vi "manual-induction-furnace-control-v5.vi"() -> ()   [LabVIEW 2019]
uses:
  <vilib>/DAQmx/read.llb/DAQmx Read (Analog 2D DBL NChan NSamp).vi
  <vilib>/Analysis/baseanly.llb/Mean (DBL).vi
  <vilib>/DAQmx/read.llb/DAQmx Read (Analog 1D DBL 1Chan NSamp).vi
  <vilib>/DAQmx/write.llb/DAQmx Write (Analog DBL 1Chan 1Samp).vi
  <vilib>/DAQmx/create/channels.llb/DAQmx Create Channel (AO-Current-Basic).vi
  <vilib>/DAQmx/create/channels.llb/DAQmx Create Channel (AI-Current-Basic).vi
  <vilib>/DAQmx/create/channels.llb/DAQmx Create Channel (AI-Voltage-Basic).vi
  <vilib>/DAQmx/miscellaneous.llb/DAQmx Fill In Error Info.vi
  <vilib>/Analysis/NI_AALBase.lvlib
panel:
  out "Error Detected":bool
  in  "Furnace Enable":bool
  in  "Furnace Stop":bool
  out "Valve Output":dbl format="%#_3g"
  in  "ESTOP":bool
  in  "Valve Open":bool
  in  "Purge Flow On":bool
  out "Pressure":dbl format="%#_3g"
  in  "Tab Control":enum32{"Start", "Test", "End"}(tab)
  in  "Start Test":bool
  out "Waveform Chart":dynamicdata(graph)
  out "Test Elapsed Time":string
  in  "Stop / Reset":bool=TRUE caption="Start"
  in  "Data Log?":bool caption="Enable"
  in  "Data Collection Rate (10 hz max)":dbl=1.0 caption="Time Target (s)"
  in  "Pressure Limit (vacuum)":dbl=770.0
  in  "Temp change limit (per 0.5 sec)":dbl=60.0
  in  "Max Temp Limit":dbl=2600.0
  in  "Error Notification Recipient emails":string[](array[string])
  in  "Furnace Power":dbl min=0.0 max=100.0 step=0.1 format="%#.1f"
  in  "Argon Out":dbl format="%#_4g"
  in  "Auto ramp to 10%":bool
  in  "Heat-up rate":enum16{"Low", "Medium", "High"}(ring)
  in  "Filename":path=path "test.lvm"
  out "End Result":string
  out "Temperature":dbl format="%#_5g"
  out "Power Out":dbl
  # "%"
  # "°C"
  # "Torr"
  # "Check all of your hardware and setup, install your sample, turn on purge gas and pump down to your desired vacuum.\n\nClick the \"Start Test\" button when you are ready to start heating."
  # "This is a manual control window. Use the Auto Ramp button to get you to ~10%, then slowly increment the power percentage from 10% to your desired power while monitoring the temperature. Between each time you increment the power, allow enough time for the item in the furnace to come to equilibrium before increasing the power more."
  # "Manual Controls"
  # "%"
  # "%"
  # "Safety Shutoff Limits"
  # "Torr"
  # "°C"
  # "°C"
  # "Your test has been stopped. Below you can see if the test finished successfully or if an error occurred."
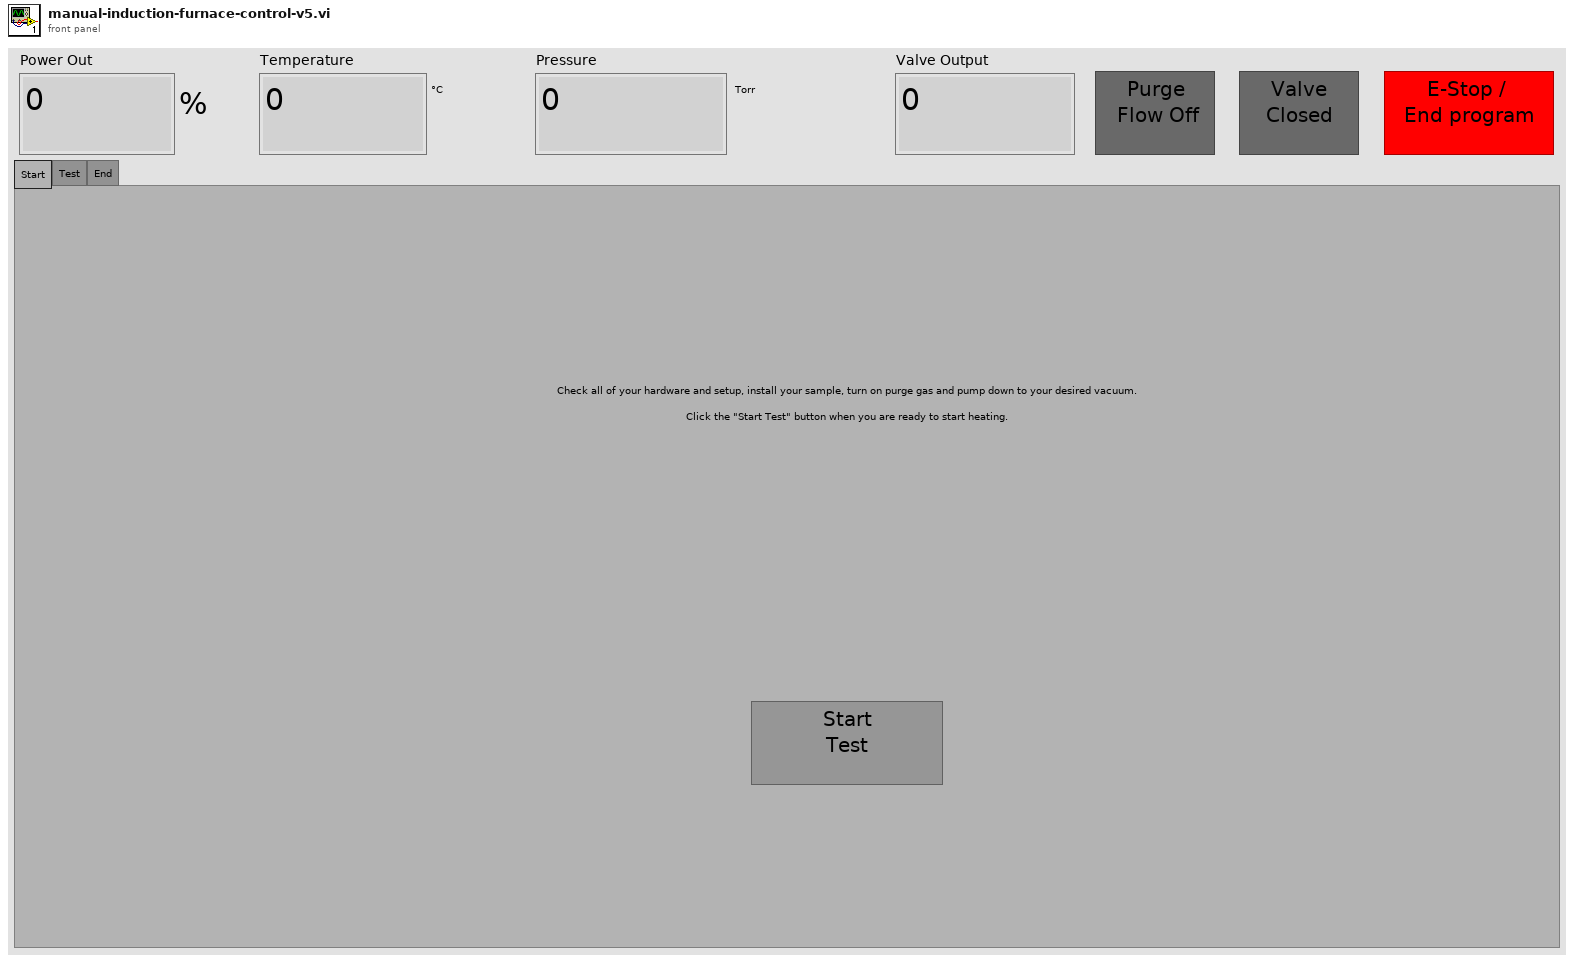
[diagram p1: front panel]
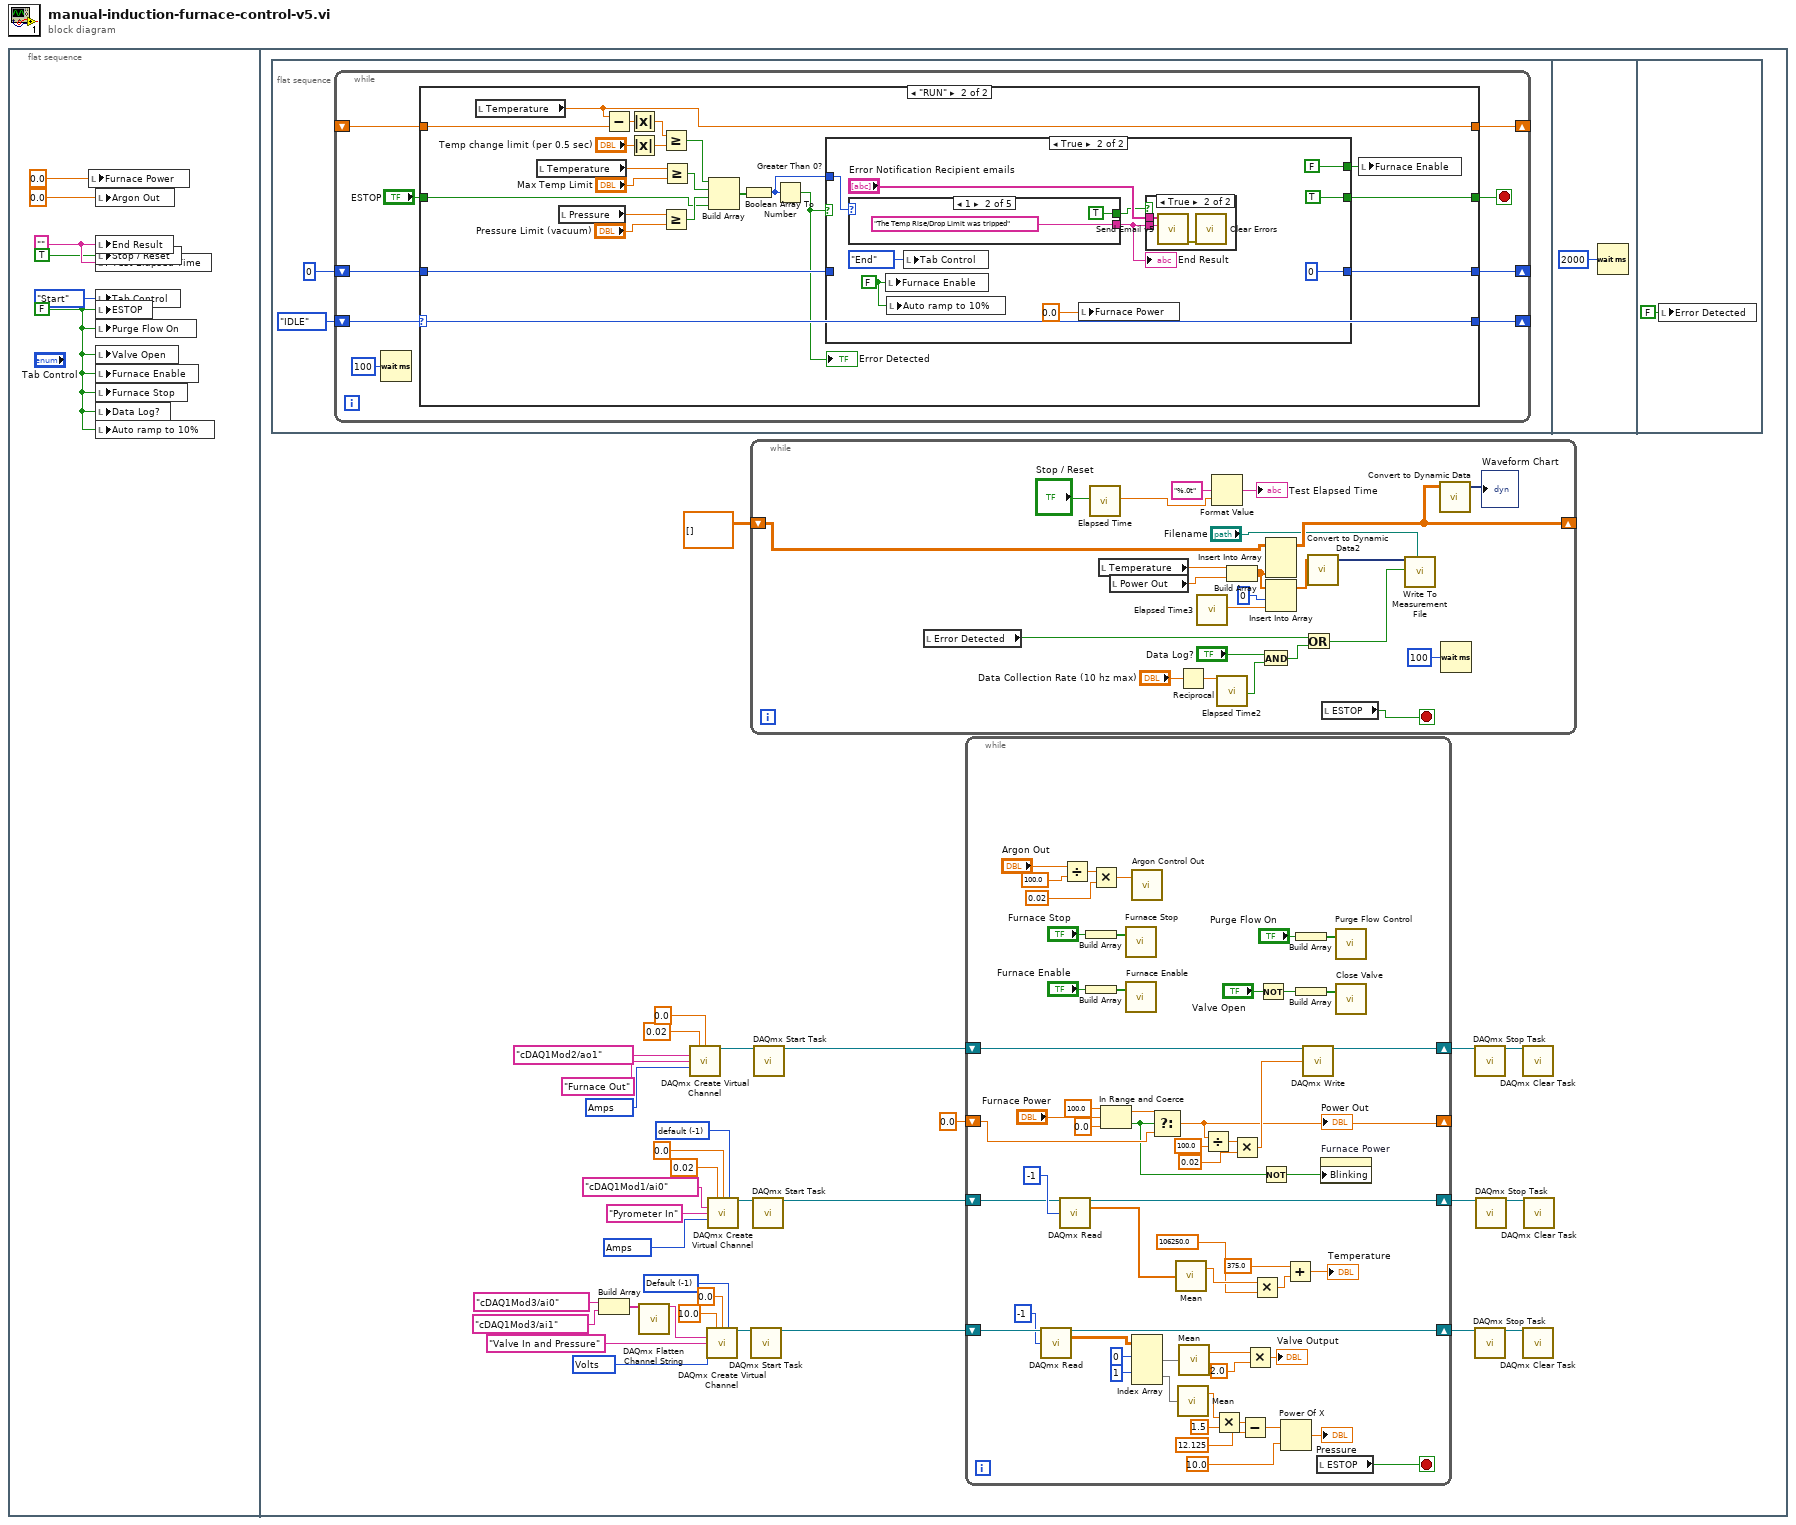
[diagram p0: block diagram]
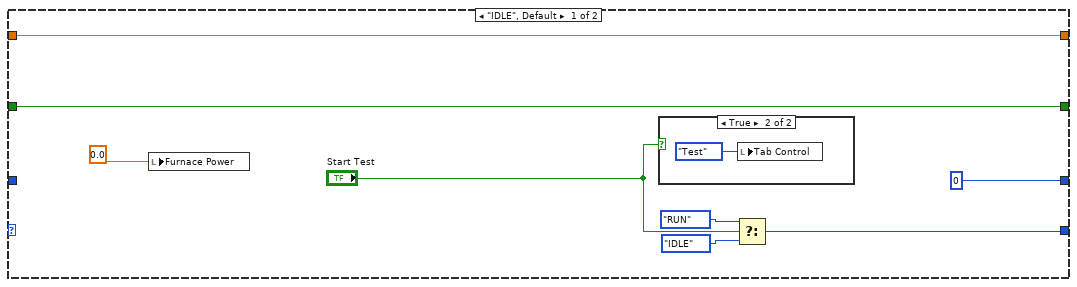
[diagram p2: hidden frame]
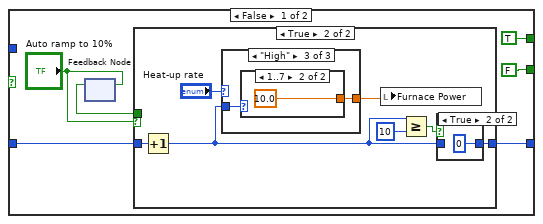
[diagram p4: hidden frame]
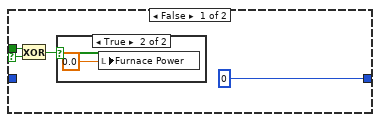
[diagram p5: hidden frame]
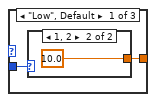
[diagram p7: hidden frame]
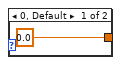
[diagram p8: hidden frame]
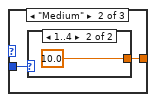
[diagram p9: hidden frame]
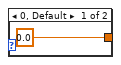
[diagram p10: hidden frame]
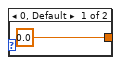
[diagram p11: hidden frame]
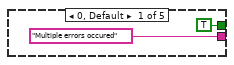
[diagram p14: hidden frame]
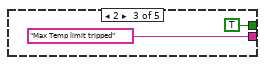
[diagram p15: hidden frame]
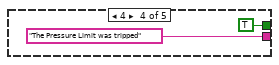
[diagram p16: hidden frame]
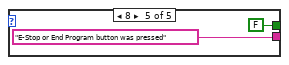
[diagram p17: hidden frame]
diagram:
  n1 = flat-sequence {
    frame #0 {
      w5 = "" ("End Result")
      w1 = FALSE
      n2 = local write "Furnace Power"(0.0 ("Power Input")) -> ()
      n3 = local write "Argon Out"(0.0 ("Pressure Limit")) -> ()
      n4 = local write "End Result"(w5) -> ()
      n5 = local write "Stop / Reset"(TRUE ("Stop / Reset")) -> ()
      n6 = local write "Test Elapsed Time"(w5) -> ()
      n7 = local write "Tab Control"(enum32{"Start", "Test", "End"}."Start" ("Tab Control")) -> ()
      n8 = local write "ESTOP"(w1) -> ()
      n9 = local write "Purge Flow On"(w1) -> ()
      n10 = local write "Valve Open"(w1) -> ()
      n11 = local write "Furnace Enable"(w1) -> ()
      n12 = local write "Furnace Stop"(w1) -> ()
      n13 = local write "Data Log?"(w1) -> ()
      n14 = local write "Auto ramp to 10%"(w1) -> ()
    }
    frame #1 {
      w20 = 10348 items=["Volts"=10348, "From Custom Scale"=10065] ("units")
      w22 = -1 items=["Default"=-1, "RSE"=10083, "NRSE"=10078, "Differential"=10106, "Pseudodifferential"=12529] ("input terminal configuration")
      w27 = -1 items=["default"=-1, "RSE"=10083, "NRSE"=10078, "Differential"=10106, "Pseudodifferential"=12529] ("input terminal configuration")
      w19 = 10342 items=["Amps"=10342, "From Custom Scale"=10065] ("units")
      w32 = 10342 items=["Amps"=10342, "From Custom Scale"=10065] ("units")
      n15 = flat-sequence {
        frame #0 {
          n16 = while {
            shift-right: [w47] -> _
            shift-left: enum16{"IDLE", "RUN"}."IDLE" -> [w49]
            shift-right: [w51] -> _
            shift-left: _ -> [w50]
            shift-right: [w45] -> _
            shift-left: 0 -> [w46]
            stop <- w43 stop-if-true
            n17 = Wait (ms)(milliseconds to wait=u32 100) -> ()  [unwired: 1 out]
            n18 = case shown="\"RUN\"" w49 {
              selector: w49 -> [_ w65]
              tunnel: [w59 w80] -> w51
              tunnel: w50 -> [w59 w79]
              tunnel: [w58 w66] -> w43
              tunnel: "ESTOP" -> [w58 w67]
              tunnel: [w55 w65] -> w47
              tunnel: w46 -> [_ w63]
              tunnel: [0 w62] -> w45
              frame "IDLE", Default {
                n19 = local write "Furnace Power"(0.0 ("Power Input")) -> ()
                n20 = case shown="True" "Start Test" {
                  frame False {
                  }
                  frame True {
                    n21 = local write "Tab Control"(enum32{"Start", "Test", "End"}."Test" ("Tab Control")) -> ()
                  }
                }
                n22 = Select(t=enum16{"IDLE", "RUN"}."RUN", s="Start Test", f=enum16{"IDLE", "RUN"}."IDLE") -> (s? t:f=w55:enum16{"IDLE", "RUN"})
              }
              frame "RUN" {
                n23 = local read "Temperature"() -> (w80:dbl)
                n24 = local read "Temperature"() -> (w74:dbl)
                n25 = local read "Pressure"() -> (w82:dbl)
                n26 = Subtract(x=w80, y=w79) -> (x-y=w76:dbl)
                n27 = Absolute Value(x=w76) -> (abs(x)=w75:dbl)
                n28 = Absolute Value(x="Temp change limit (per 0.5 sec)") -> (abs(x)=w77:dbl)
                n29 = Greater Or Equal?(x=w75, y=w77) -> (x >= y?=w72:bool)
                n30 = Greater Or Equal?(x=w82, y="Pressure Limit (vacuum)") -> (x >= y?=w70:bool)
                n31 = Greater Or Equal?(x=w74, y="Max Temp Limit") -> (x >= y?=w71:bool)
                n32 = Build Array(w72, w71, w70, w67) -> (w69:bool[])
                n33 = Boolean Array To Number(Boolean array=w69) -> (number=w68:u32)
                n34 = Greater Than 0?(x=w68) -> (x > 0?=w61:bool)
                "Error Detected" <- w61
                n35 = case shown="True" w61 {
                  tunnel: w68 -> [_ w123]
                  tunnel: [FALSE TRUE] -> w66
                  tunnel: [TRUE ("Furnace Enable") FALSE ("Furnace Enable")] -> w64
                  tunnel: w63 -> [w86 _]
                  tunnel: [w85 0] -> w62
                  frame False {
                    n36 = feedback #1() -> (w83:bool)  [unwired: 1 in]
                    n37 = feedback-in #1("Auto ramp to 10%") -> ()
                    n38 = case shown="True" "Auto ramp to 10%" {
                      selector: "Auto ramp to 10%" -> [w91 _]
                      tunnel: w86 -> [_ w100]
                      tunnel: [0 w99] -> w85
                      tunnel: w83 -> [w89 _]
                      frame False {
                        n39 = Exclusive Or(1:w91, 2:w89) -> (0:w90:bool)
                        n40 = case shown="True" w90 {
                          frame False {
                          }
                          frame True {
                            n41 = local write "Furnace Power"(0.0) -> ()
                          }
                        }
                      }
                      frame True {
                        n42 = Increment(x=w100) -> (x+1=w95:i32)
                        n43 = case shown="\"High\"" "Heat-up rate" {
                          tunnel: w95 -> [w102 w106 w110]
                          tunnel: [w101 w105 w109] -> w94
                          frame "Low", Default {
                            n44 = case shown="1, 2" w102 {
                              tunnel: [0.0 10.0] -> w101
                              frame 0, Default {
                              }
                              frame 1, 2 {
                              }
                            }
                          }
                          frame "Medium" {
                            n45 = case shown="1..4" w106 {
                              tunnel: [0.0 10.0] -> w105
                              frame 0, Default {
                              }
                              frame 1..4 {
                              }
                            }
                          }
                          frame "High" {
                            n46 = case shown="1..7" w110 {
                              tunnel: [0.0 10.0] -> w109
                              frame 0, Default {
                              }
                              frame 1..7 {
                              }
                            }
                          }
                        }
                        n47 = local write "Furnace Power"(w94) -> ()
                        n48 = Greater Or Equal?(x=w95, y=10) -> (x >= y?=w97:bool)
                        n49 = case shown="True" w97 {
                          tunnel: w95 -> [w113 _]
                          tunnel: [w113 0] -> w99
                          frame False {
                          }
                          frame True {
                          }
                        }
                      }
                    }
                  }
                  frame True {
                    w115 = FALSE ("Furnace Enable")
                    n50 = case shown="1" w123 {
                      tunnel: ["Multiple errors occured" ("End Result") "The Temp Rise/Drop Limit was tripped" ("End Result") "Max Temp limit tripped" ("End Result") "The Pressure Limit was tripped" ("End Result") "E-Stop or End Program button was pressed" ("End Result")] -> w122
                      tunnel: [TRUE ("Furnace Enable") TRUE ("Furnace Enable") TRUE ("Furnace Enable") TRUE ("Furnace Enable") FALSE ("Furnace Enable")] -> w120
                      frame 0, Default {
                      }
                      frame 1 {
                      }
                      frame 2 {
                      }
                      frame 4 {
                      }
                      frame 8 {
                      }
                    }
                    "End Result" <- w122
                    n51 = local write "Furnace Enable"(w115) -> ()
                    n52 = local write "Auto ramp to 10%"(w115) -> ()
                    n53 = local write "Tab Control"(enum32{"Start", "Test", "End"}."End" ("Tab Control")) -> ()
                    n54 = local write "Furnace Power"(0.0) -> ()
                    n55 = case shown="True" w120 {
                      tunnel: "Error Notification Recipient emails" -> [_ w126]
                      tunnel: w122 -> [_ w125]
                      frame False {
                      }
                      frame True {
                        n56 = call "Send Email v5.vi"("Message"=w125, "Recipient emails"=w126) -> ("error out"=w127:errorcluster)  [unwired: 9 in]
                        n57 = call <vilib>:"Clear Errors.vi"("error in (no error)"=w127) -> ()  [unwired: 5 in, 2 out]
                      }
                    }
                  }
                }
                n58 = local write "Furnace Enable"(w64) -> ()
              }
            }
          }
        }
        frame #1 {
          n59 = Wait (ms)(milliseconds to wait=u32 2000) -> ()  [unwired: 1 out]
        }
        frame #2 {
          n60 = local write "Error Detected"(FALSE ("Error Detected")) -> ()
        }
      }
      n61 = Build Array(tag "cDAQ1Mod3/ai0" ("physical channels"), tag "cDAQ1Mod3/ai1" ("physical channels")) -> (w16:tag[])
      n62 = call <vilib>:"DAQmx Flatten Channel String.vi"("names in"=w16) -> ("names out"=w15:string)  [unwired: 13 in, 1 out]
      n63 = call-poly <vilib>:"DAQmx Create Virtual Channel.vi"("maximum value"=0.02, "minimum value"=0.0, "physical channels"=tag "cDAQ1Mod2/ao1", "name to assign"="Furnace Out", "units"=w32) -> ("task out"=w33:refnum<k21>)  [unwired: 9 in, 1 out]
      n64 = call-poly <vilib>:"DAQmx Create Virtual Channel.vi"("maximum value"=10.0, "minimum value"=0.0, "input terminal configuration"=w22, "physical channels"=w15, "name to assign"="Valve In and Pressure", "units"=w20) -> ("task out"=w25:refnum<k21>)  [unwired: 8 in, 1 out]
      n65 = call-poly <vilib>:"DAQmx Create Virtual Channel.vi"("maximum value"=0.02, "minimum value"=0.0, "input terminal configuration"=w27, "physical channels"=tag "cDAQ1Mod1/ai0", "name to assign"="Pyrometer In", "units"=w19) -> ("task out"=w26:refnum<k21>)  [unwired: 8 in, 1 out]
      n66 = while {
        shift-right: [w142] -> _
        shift-left: dbl[][] [] -> [w144]
        stop <- w163 stop-if-true
        n67 = local read "Error Detected"() -> (w145:bool)
        n68 = call "Elapsed Time"("Reset"="Stop / Reset") -> ("Elapsed Time (s)"=w161:dbl)  [unwired: 11 in, 7 out]
        n69 = local read "Temperature"() -> (w155:dbl)
        n70 = local read "Power Out"() -> (w156:dbl)
        n71 = Reciprocal(x="Data Collection Rate (10 hz max)") -> (1/x=w148:dbl)
        n72 = call "Elapsed Time3"() -> ("Elapsed Time (s)"=w152:dbl)  [unwired: 12 in, 7 out]
        n73 = Format Value(format string="%.0t", value (0)=w161) -> (output string=→"Test Elapsed Time":string)  [unwired: 1 in]
        n74 = call "Elapsed Time2"("Time Target (s)"=w148) -> ("Time has Elapsed"=w154:bool)  [unwired: 11 in, 7 out]
        n75 = Build Array(w155, w156) -> (w150:dbl[])
        n76 = And(x="Data Log?", y=w154) -> (x .and. y?=w157:bool)
        n77 = Insert Into Array(array=w144, new element=w150) -> (w142:dbl[][])  [unwired: 2 in]
        n78 = Insert Into Array(array=w150, index=0, new element=w152) -> (w151:dbl[])
        n79 = Or(x=w145, y=w157) -> (x .or. y?=w158:bool)
        n80 = call "Convert to Dynamic Data2"("Array"=w151) -> ("Dynamic Data Type"=w149:dynamicdata)  [unwired: 3 in]
        n81 = local read "ESTOP"() -> (w163:bool)
        n82 = call "Write To Measurement File"("Signals"=w149, "Enable"=w158, "Filename"="Filename") -> ()  [unwired: 14 in, 3 out]
        n83 = call "Convert to Dynamic Data"("2D Array"=w142) -> ("Dynamic Data Type"=→"Waveform Chart":dynamicdata)  [unwired: 3 in]
        n84 = Wait (ms)(milliseconds to wait=u32 100) -> ()  [unwired: 1 out]
      }
      n85 = call <vilib>:"DAQmx Start Task.vi"("task/channels in"=w25) -> ("task out"=w38:refnum<k21>)  [unwired: 13 in, 1 out]
      n86 = call <vilib>:"DAQmx Start Task.vi"("task/channels in"=w26) -> ("task out"=w40:refnum<k21>)  [unwired: 13 in, 1 out]
      n87 = call <vilib>:"DAQmx Start Task.vi"("task/channels in"=w33) -> ("task out"=w39:refnum<k21>)  [unwired: 13 in, 1 out]
      n88 = while {
        shift-right: [w197] -> w11
        shift-left: w39 -> [w199]
        shift-right: [w200] -> w13
        shift-left: w40 -> [w202]
        shift-right: [w193] -> w9
        shift-left: w38 -> [w195]
        shift-right: [w164] -> _
        shift-left: 0.0 ("upper limit") -> [w167]
        stop <- w172 stop-if-true
        n89 = call-poly <vilib>:"DAQmx Read.vi"("task/channels in"=w195, "number of samples per channel"=-1) -> ("task out"=w193:refnum<k21>, "data"=w184:dbl[][])  [unwired: 11 in, 1 out]
        n90 = call-poly <vilib>:"DAQmx Read.vi"("task/channels in"=w202, "number of samples per channel"=-1) -> ("task out"=w200:refnum<k21>, "data"=w203:dbl[])  [unwired: 11 in, 1 out]
        n91 = Divide(x="Argon Out", y=100.0) -> (x/y=w177:dbl)
        n92 = Build Array("Furnace Stop") -> (w215:bool[])
        n93 = Build Array("Furnace Enable") -> (w216:bool[])
        n94 = Multiply(x=w177, y=0.02) -> (x*y=w173:dbl)
        n95 = In Range and Coerce(upper limit=100.0, x="Furnace Power", lower limit=0.0) -> (coerced(x)=w168:dbl, In Range?=w166:bool)
        n96 = call "Furnace Stop"("data"=w215) -> ()  [unwired: 17 in, 2 out]
        n97 = call "Furnace Enable"("data"=w216) -> ()  [unwired: 17 in, 2 out]
        n98 = call "Argon Control Out"("data"=w173) -> ()  [unwired: 17 in, 2 out]
        n99 = Index Array(array=w184, index (row) #1=0 ("index (row)"), index (row) #2=1 ("index (row)")) -> (element #1=w181:dbl[], element #2=w180:dbl[])  [unwired: 2 in]
        n100 = Select(t=w168, s=w166, f=w167) -> (s? t:f=w164:dbl)
        "Power Out" <- w164
        n101 = call-poly <vilib>:"Mean.vi"("X"=w203) -> ("mean"=w207:dbl)  [unwired: 1 out]
        n102 = call-poly <vilib>:"Mean.vi"("X"=w180) -> ("mean"=w192:dbl)  [unwired: 1 out]
        n103 = call-poly <vilib>:"Mean.vi"("X"=w181) -> ("mean"=w185:dbl)  [unwired: 1 out]
        n104 = Divide(x=w164, y=100.0) -> (x/y=w210:dbl)
        n105 = Multiply(x=w192, y=1.5) -> (x*y=w190:dbl)
        n106 = Multiply(x=w210, y=0.02) -> (x*y=w198:dbl)
        n107 = Subtract(x=w190, y=12.125) -> (x-y=w188:dbl)
        n108 = Multiply(x=w185, y=2.0) -> (x*y=→"Valve Output":dbl)
        n109 = Multiply(x=w207, y=106250.0) -> (x*y=w206:dbl)
        n110 = Not(x="Valve Open") -> (.not. x?=w178:bool)
        n111 = Not(x=w166) -> (.not. x?=w165:bool)
        n112 = Power Of X(1:10.0 ("x"), 2:w188) -> (0:→"Pressure":dbl)
        n113 = Add(x=375.0, y=w206) -> (x+y=→"Temperature":dbl)
        n114 = Build Array("Purge Flow On") -> (w213:bool[])
        n115 = Build Array(w178) -> (w212:bool[])
        n116 = call-poly <vilib>:"DAQmx Write.vi"("task/channels in"=w199, "data"=w198) -> ("task out"=w197:refnum<k21>)  [unwired: 11 in, 2 out]
        n117 = local read "ESTOP"() -> (w172:bool)
        n118 = property on="Furnace Power" class="DigNum (strict)"("Blinking"=w165) -> ()  [unwired: 2 in, 2 out]
        n119 = call "Purge Flow Control"("data"=w213) -> ()  [unwired: 17 in, 2 out]
        n120 = call "Close Valve"("data"=w212) -> ()  [unwired: 17 in, 2 out]
      }
      n121 = call <vilib>:"DAQmx Stop Task.vi"("task/channels in"=w11) -> ("task out"=w12:refnum<k21>)  [unwired: 13 in, 1 out]
      n122 = call <vilib>:"DAQmx Stop Task.vi"("task/channels in"=w9) -> ("task out"=w10:refnum<k21>)  [unwired: 13 in, 1 out]
      n123 = call <vilib>:"DAQmx Stop Task.vi"("task/channels in"=w13) -> ("task out"=w14:refnum<k21>)  [unwired: 13 in, 1 out]
      n124 = call <vilib>:"DAQmx Clear Task.vi"("task in"=w12) -> ()  [unwired: 14 in, 1 out]
      n125 = call <vilib>:"DAQmx Clear Task.vi"("task in"=w10) -> ()  [unwired: 14 in, 1 out]
      n126 = call <vilib>:"DAQmx Clear Task.vi"("task in"=w14) -> ()  [unwired: 14 in, 1 out]
    }
  }
